vi "search for com resources.vi"(8 "error in (no error)":errorcluster) -> (0 "error out":errorcluster, 1 "Number of Com Ports Present in System > 0?":bool, 2 "Number of Com Ports Present in System":i32, 3 "List of Com Ports Present in System":refnum<visa-resource-name>[](array[refnum]))   [LabVIEW 2016]
uses:
  <vilib>/Instr/_visa.llb/VISA Find Search Mode.ctl
panel:
  out "Array":errorcluster[](array[cluster])
  out "List of COM Ports":string[](array[string])
  out "find list":string[](array[string])
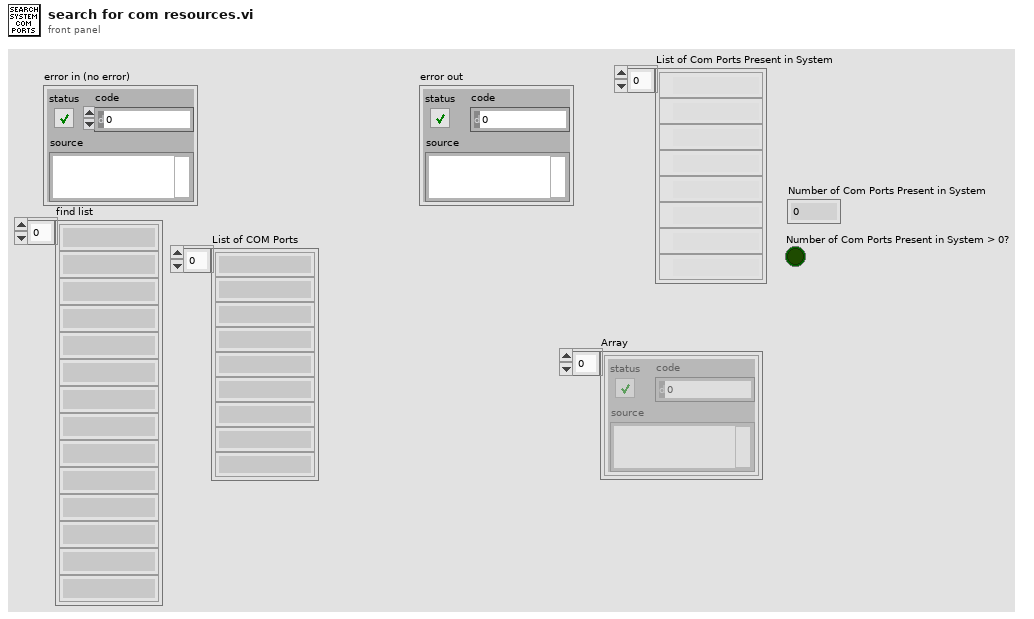
[diagram p1: front panel]
types:
  T1 = typedef "VISA Find Search Mode.ctl" = u32
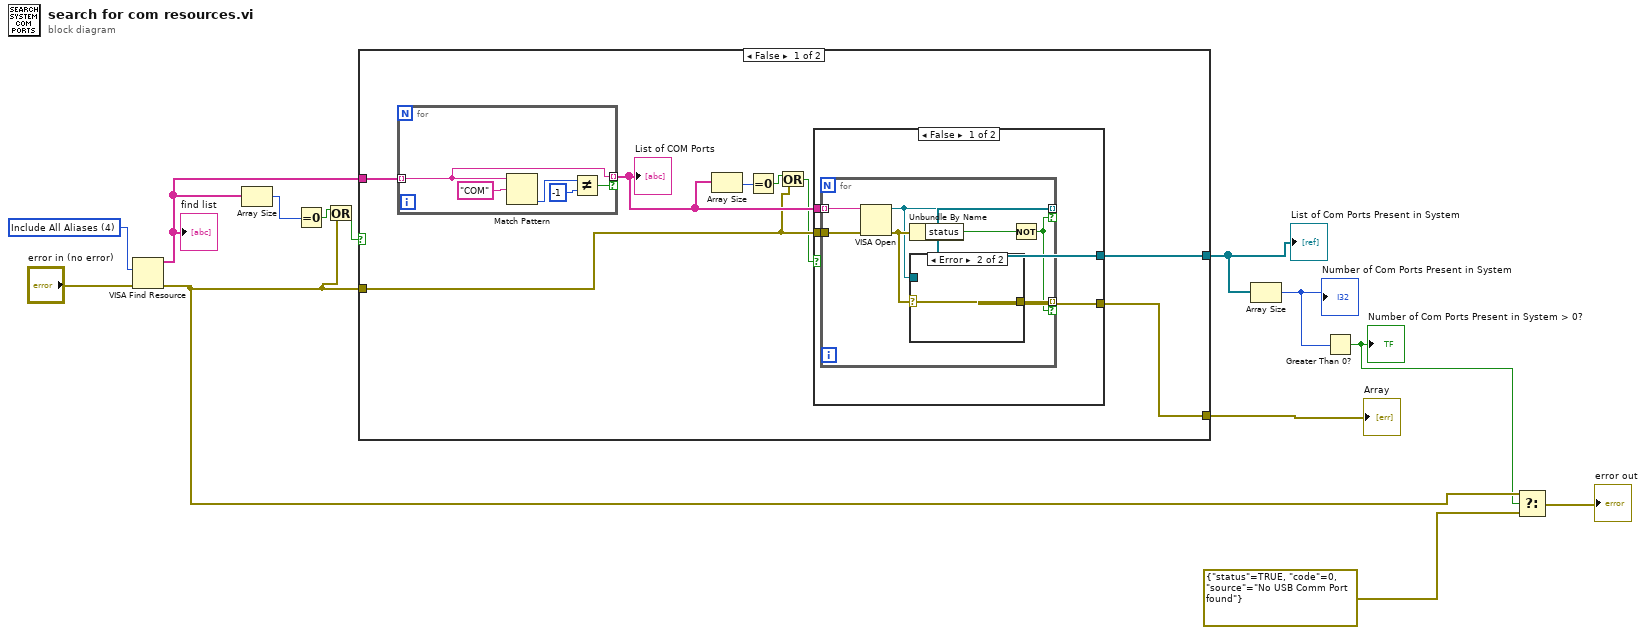
[diagram p0: block diagram]
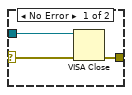
[diagram p2: hidden frame]
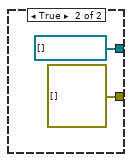
[diagram p3: hidden frame]
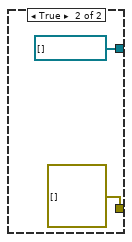
[diagram p4: hidden frame]
diagram:
  w12 = T1 4 items=["Canonical Names Only"=0, "Aliases Only"=2, "Include Matching Aliases"=3, "Include All Aliases"=4] ("Search Mode")
  n1 = VISA Find Resource(8:"error in (no error)", 10:w12) -> (0:w3:errorcluster, 3:w11:string[])  [unwired: 1 in, 1 out]
  "find list" <- w11
  n2 = Array Size(array=w11) -> (size(s)=w10:i32)
  n3 = Equal To 0?(x=w10) -> (x = 0?=w5:bool)
  n4 = Or(x=w5, y=w3) -> (x .or. y?=w7:bool)
  n5 = case shown="False" w7 {
    tunnel: w3 -> [w15 _]
    tunnel: w11 -> [w21 _]
    tunnel: [w20 refnum<visa-resource-name>[] []] -> w9
    tunnel: [w19 errorcluster[] []] -> w6
    frame False {
      n6 = for {
        tunnel: w21 -> [w40] mode=indexing
        tunnel: [w40] -> w18 mode=indexing if=w39
        n7 = Match Pattern(string=w40, regular expression="COM") -> (offset past match=w42:i32)  [unwired: 1 in, 3 out]
        n8 = Not Equal?(x=w42, y=-1) -> (x != y?=w39:bool)
      }
      "List of COM Ports" <- w18
      n9 = Array Size(array=w18) -> (size(s)=w17:i32)
      n10 = Equal To 0?(x=w17) -> (x = 0?=w16:bool)
      n11 = Or(x=w16, y=w15) -> (x .or. y?=w14:bool)
      n12 = case shown="False" w14 {
        tunnel: [w25 refnum<visa-resource-name>[] []] -> w20
        tunnel: [w24 errorcluster[] []] -> w19
        tunnel: w18 -> [w23 _]
        tunnel: w15 -> [w22 _]
        frame False {
          n13 = for {
            tunnel: w22 -> [w32]
            tunnel: w23 -> [w31] mode=indexing
            tunnel: [w28] -> w25 mode=indexing if=w26
            tunnel: [w27] -> w24 mode=indexing if=w26
            n14 = VISA Open(error in (no error)=w32, VISA resource name=w31) -> (VISA resource name=w28:refnum<visa-resource-name>, error out=w29:errorcluster)  [unwired: 3 in]
            n15 = Unbundle By Name(w29) -> ("status"=w30:bool)
            n16 = case shown="Error" w29 {
              selector: w29 -> [w34 w36]
              tunnel: w28 -> [w35 _]
              tunnel: [w33 w36] -> w27
              frame No Error {
                n17 = VISA Close(VISA resource name=w35, error in (no error)=w34) -> (error out=w33:errorcluster)
              }
              frame Error {
              }
            }
            n18 = Not(x=w30) -> (.not. x?=w26:bool)
          }
        }
        frame True {
        }
      }
    }
    frame True {
    }
  }
  "List of Com Ports Present in System" <- w9
  "Array" <- w6
  n19 = Array Size(array=w9) -> (size(s)=w8:i32)
  "Number of Com Ports Present in System" <- w8
  n20 = Greater Than 0?(x=w8) -> (x > 0?=w2:bool)
  "Number of Com Ports Present in System > 0?" <- w2
  n21 = Select(t=w3, s=w2, f=errorcluster {"status"=TRUE, "code"=0, "source"="No USB Comm Port found"}) -> (s? t:f=→"error out":errorcluster)
